vi "Find Ball.vi"(8 "Error In":errorcluster, 11 "Ball Object":T1) -> (0 "Error Out":errorcluster)   [LabVIEW 2018]
uses:
  Image Object.ctl
  Ball Data.vi
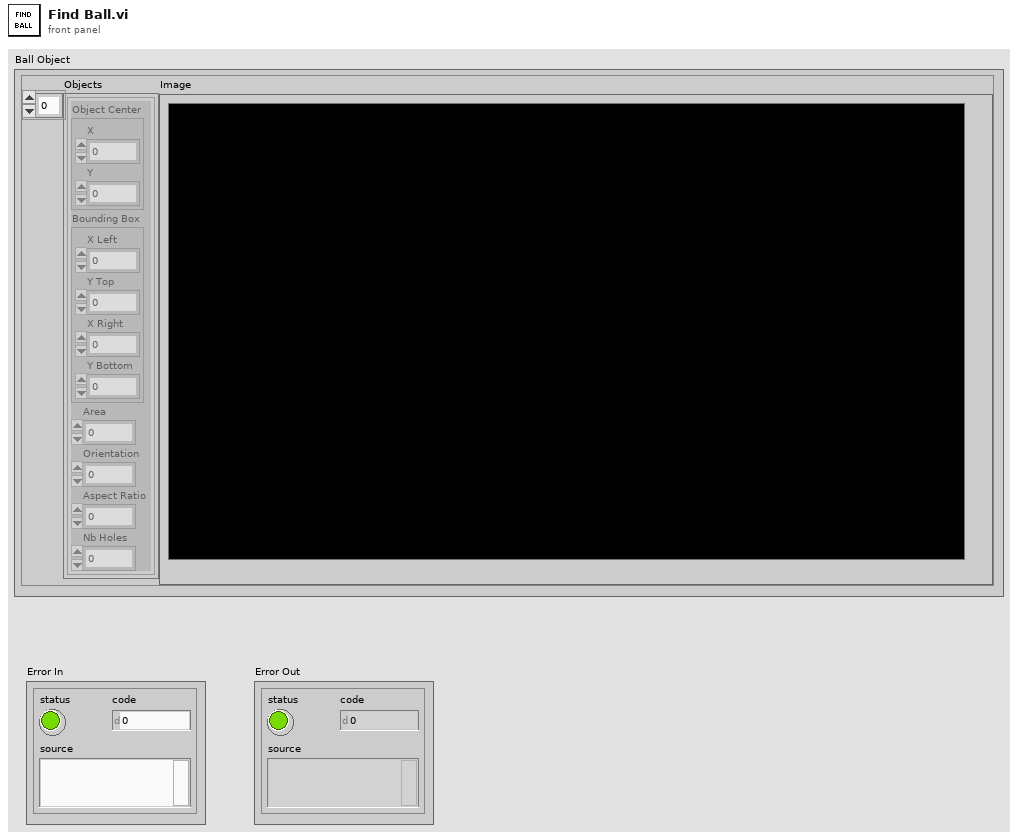
[diagram p1: front panel]
types:
  T1 = typedef "Image Object.ctl" = cluster{"Objects":cluster{"Object Center":cluster{"X":sgl, "Y":sgl}, "Bounding Box":cluster{"X Left":i32, "Y Top":i32, "X Right":i32, "Y Bottom":i32}, "Area":sgl, "Orientation":sgl, "Aspect Ratio":sgl, "Nb Holes":i32}[], "Image":T2}
  T2 = typedef "IMAQ Image.ctl" = refnum<image>
  T3 = cluster{"Object Center":cluster{"X":sgl, "Y":sgl}, "Bounding Box":cluster{"X Left":i32, "Y Top":i32, "X Right":i32, "Y Bottom":i32}, "Area":sgl, "Orientation":sgl, "Aspect Ratio":sgl, "Nb Holes":i32}[]
  T4 = cluster{"Object Center":cluster{"X":sgl, "Y":sgl}, "Bounding Box":cluster{"X Left":i32, "Y Top":i32, "X Right":i32, "Y Bottom":i32}, "Area":sgl, "Orientation":sgl, "Aspect Ratio":sgl, "Nb Holes":i32}
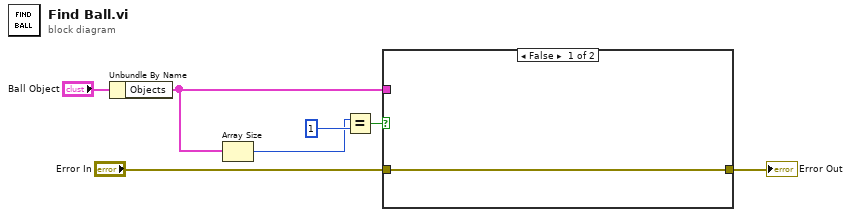
[diagram p0: block diagram]
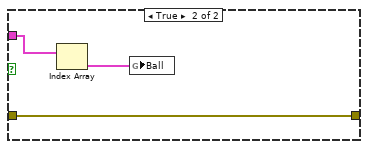
[diagram p2: hidden frame]
diagram:
  n1 = Unbundle By Name("Ball Object") -> ("Objects"=w3:T3)
  n2 = Array Size(array=w3) -> (size(s)=w4:i32)
  n3 = Equal?(x=w4, y=1) -> (x = y?=w6:bool)
  n4 = case shown="False" w6 {
    tunnel: w3 -> [_ w11]
    tunnel: "Error In" -> [w8 w9]
    tunnel: [w8 w9] -> w1
    frame False {
    }
    frame True {
      n5 = Index Array(array=w11) -> (element=w10:T4)  [unwired: 1 in]
      n6 = global write "Ball Data.vi" "Ball"(w10) -> ()
    }
  }
  "Error Out" <- w1
